vi "Config.vi"() -> ()   [LabVIEW 2014, in "Daqmx Module tests.lvlib"]
uses:
  Daqmx Module tests.lvlib
  <resource>/objmgr/daqmx.rc
panel:
  out "Real Device Product Types":string[](array[string])
  out "BusType":i32[](array[ring]) items=["PCI"=12582, "PCIe"=13612, "PXI"=12583, "PXIe"=14706, "SCXI"=12584, "SCC"=14707, "PCCard"=12585, "USB"=12586, "CompactDAQ"=14637, "TCP/IP"=14828, "Unknown"=12588, "SwitchBlock"=15870]
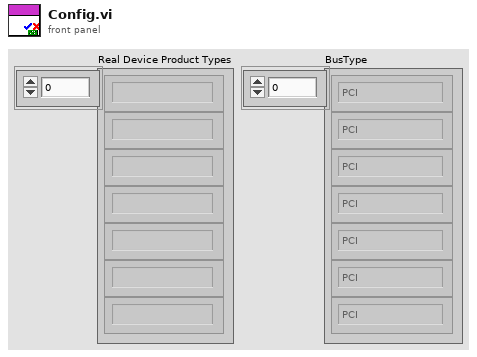
[diagram p1: front panel]
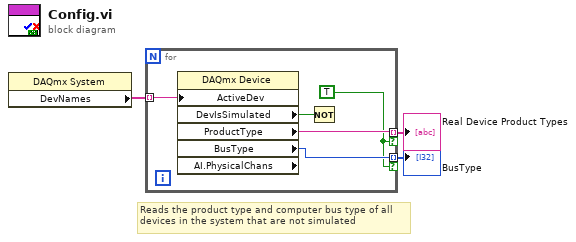
[diagram p0: block diagram]
diagram:
  # "Reads the product type and computer bus type of all devices in the system that are not simulated"
  n1 = property class="DAQmx System"() -> ("DevNames"=w3:tag[])  [unwired: 2 in, 2 out]
  n2 = for {
    tunnel: w3 -> [w8] mode=indexing
    tunnel: [w7] -> w2 mode=indexing if=w4
    tunnel: [w6] -> w1 mode=indexing if=w4
    w4 = TRUE (".not. x?")
    (unwired) FALSE
    n3 = property class="DAQmx Device" props=["ActiveDev", "DevIsSimulated", "ProductType", "BusType", "AI.PhysicalChans"]("ActiveDev"=w8) -> ("DevIsSimulated"=w5:bool, "ProductType"=w7:string, "BusType"=w6:i32)  [unwired: 2 in, 3 out]
    n4 = Not(x=w5) -> ()  [unwired: 1 out]
  }
  "Real Device Product Types" <- w2
  "BusType" <- w1
